vi "construct.vi"(8 "error in (no error)":errorcluster, 9 "configuration name":string, 10 "load config file?":bool=TRUE, 11 "DL090216Display in":refnum<class "DisplayDL090216.lvclass">) -> (0 "error out":errorcluster, 3 "DL090216Display out":refnum<class "DisplayDL090216.lvclass">)   [LabVIEW 2010, in "DisplayDL090216.lvclass"]
uses:
  DisplayDL090216.lvclass
  GenericDisplay/GenericDisplay/GenericDisplay.lvclass
  DisplayDL090216.lvclass/DisplayDL090216.ctl
  ImageProcessor/ImageProcessorDL090216RangeOffset/ImageProcessorDL090216RangeOffset/ImageProcessorDL090216RangeOffset.lvclass
  ImageProcessor/GenericImageProcessor/GenericImageProcessor/GenericImageProcessor.lvclass
  common/classes/ErrorController/ErrorController/class_data.vi
  common/classes/GenericComponent/GenericComponent/GenericComponent.lvclass
  common/classes/ErrorController/ErrorController/ErrorController.lvclass
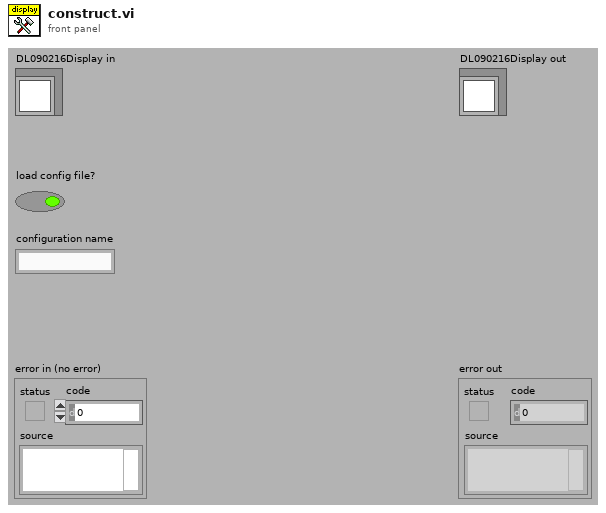
[diagram p1: front panel]
types:
  T1 = typedef "plugin_specification.ctl" = cluster{"class path":string, "configuration":string, "label":string, "settings name":string}
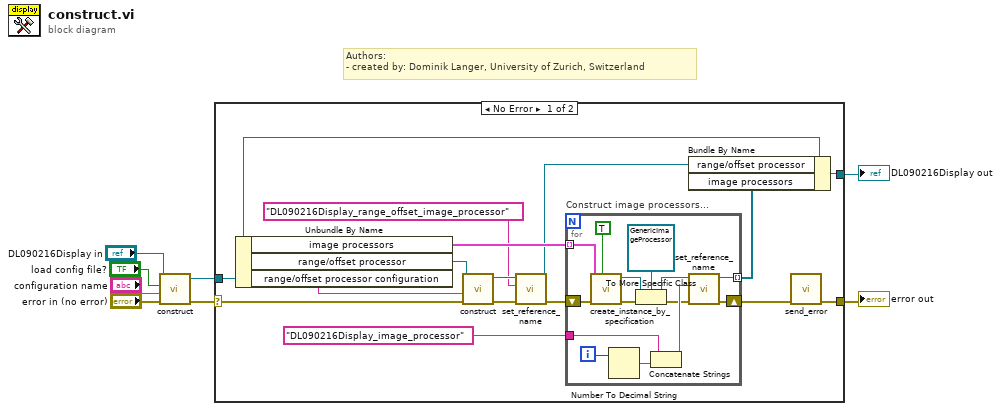
[diagram p0: block diagram]
diagram:
  # "Authors: \n- created by: Dominik Langer, University of Zurich, Switzerland"
  n1 = call-parent "construct.vi"("error in (no error)"="error in (no error)", "configuration name"="configuration name", "load config file?"="load config file?", "GenericPlugin in"="DL090216Display in") -> ("error out"=w5:errorcluster, "GenericPlugin out"=w3:refnum<class "DisplayDL090216.lvclass">)  [unwired: 6 out]
  n2 = case shown="No Error" w5 {
    selector: w5 -> [w21 w39]
    tunnel: [w9 w39] -> w8
    tunnel: [w17 w38] -> w7
    tunnel: w3 -> [w18 w38]
    frame No Error {
      n3 = Unbundle By Name(w18) -> ("image processors"=w20:T1[], "range/offset processor"=w23:refnum<class "ImageProcessorDL090216RangeOffset.lvclass">, "range/offset processor configuration"=w22:string)
      n4 = call-dynamic "construct.vi"("error in (no error)"=w21, "configuration name"=w22, "GenericPlugin in"=w23) -> ("error out"=w16:errorcluster, "GenericPlugin out"=w15:refnum<class "ImageProcessorDL090216RangeOffset.lvclass">)  [unwired: 1 in, 6 out]
      n5 = call "set_reference_name.vi"("error in (no error)"=w16, "reference name"="DL090216Display_range_offset_image_processor", "GenericPlugin.lvclass in"=w15) -> ("error out"=w12:errorcluster, "GenericPlugin.lvclass out"=w11:refnum<class "ImageProcessorDL090216RangeOffset.lvclass">)  [unwired: 7 in]
      n6 = for "Construct image processors..." {
        tunnel: w20 -> [w30] mode=indexing
        shift-right: [w33] -> w10
        shift-left: w12 -> [w31]
        tunnel: [w32] -> w19 mode=indexing
        tunnel: "DL090216Display_image_processor" -> [w35]
        i -> [w37]
        n7 = call "create_instance_by_specification.vi"("call constructor?"=TRUE, "error in (no error)"=w31, "component specification"=w30) -> ("error out"=w26:errorcluster, "GenericPlugin out"=w28:refnum<class "GenericComponent.lvclass">)  [unwired: 6 in, 1 out]
        n8 = Number To Decimal String(number=w37) -> (decimal integer string=w36:string)  [unwired: 1 out]
        n9 = To More Specific Class(target class=refnum<class "GenericImageProcessor.lvclass"> refnum ("GenericImageProcessor.lvclass"), reference=w28, error in=w26) -> (specific class reference=w27:refnum<class "GenericImageProcessor.lvclass">, error out=w25:errorcluster)
        n10 = Concatenate Strings(w35, w36) -> (w34:string)
        n11 = call "set_reference_name.vi"("error in (no error)"=w25, "reference name"=w34, "GenericPlugin.lvclass in"=w27) -> ("error out"=w33:errorcluster, "GenericPlugin.lvclass out"=w32:refnum<class "GenericImageProcessor.lvclass">)  [unwired: 7 in]
      }
      n12 = Bundle By Name(cluster=w18, "range/offset processor"=w11, "image processors"=w19) -> (w17:refnum<class "DisplayDL090216.lvclass">)
      n13 = call "send_error.vi"("error in (no error)"=w10) -> ("error out"=w9:errorcluster)  [unwired: 10 in]
    }
    frame Error {
    }
  }
  "error out" <- w8
  "DL090216Display out" <- w7
